vi "Test Next Shows Next Test to Run in Nested Test Suite.vi"(8 "error in (no error)":errorcluster, 11 "Test Case In":refnum<class "Test Suite Enumeration Test.lvclass">) -> (0 "error out":errorcluster, 3 "Test Case Out":refnum<class "Test Suite Enumeration Test.lvclass">)   [LabVIEW 2020, in "Test Suite Enumeration Test.lvclass"]
uses:
  Test Suite Enumeration Test.lvclass
  C:/Program Files (x86)/National Instruments/LabVIEW 2020/vi.lib/Astemes/LUnit/Test Case.lvclass
  Test Doubles/Test Case Test Double Child/Light Test Case Double.lvclass
  <vilib>/Astemes/LUnit/Test Case.lvclass/Test Case.ctl
  5f927c59-24be-4863-9429-5897c17c8022.vi
  <vilib>/Astemes/LUnit/Core/LUnit Test Case/Private/Append Pass Result.vi
  <vilib>/Astemes/LUnit/Core/LUnit Test Case/Private/Append Fail Result.vi
  5f927c59-24be-4863-9429-5897c17c8022.vi/9c5d11cd-9439-4240-a1ee-d9baace9c924.vi
  <vilib>/Astemes/LUnit/Core/LUnit Test Case/Private/Run In UI.vi
  <vilib>/Utility/error.llb/Clear Errors.vi
  source/Core/LUnit Test Suite/LUnit Test Suite.lvclass
  C:/git/astemes-lunit/source/Core/Runnable/Runnable.lvclass
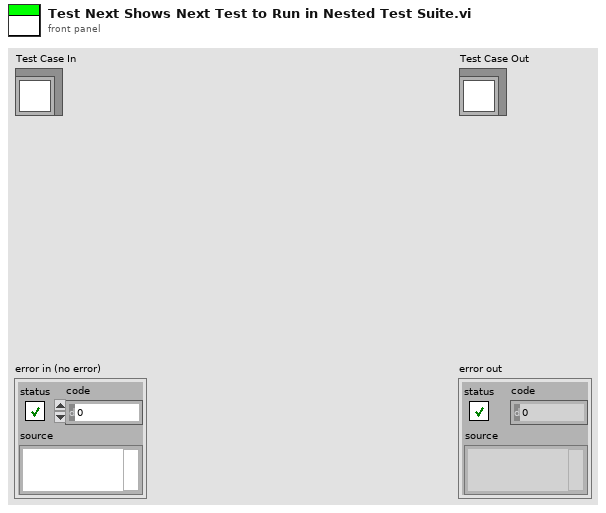
[diagram p1: front panel]
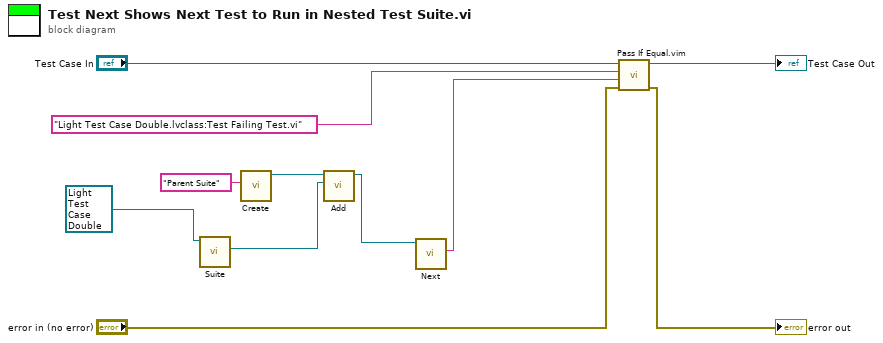
[diagram p0: block diagram]
diagram:
  n1 = call-dynamic "Suite.vi"("LUnit Test Case In"=refnum<class "Light Test Case Double.lvclass"> refnum ("Light Test Case Double.lvclass")) -> ("LUnit Test Suite Out"=w3:refnum<class "LUnit Test Suite.lvclass">)  [unwired: 8 in, 2 out]
  n2 = call "Create.vi"("Suite Name"="Parent Suite") -> ("LUnit Test Suite Out"=w4:refnum<class "LUnit Test Suite.lvclass">)  [unwired: 9 in, 1 out]
  n3 = call "Add.vi"("Runnable"=w3, "LUnit Test Suite In"=w4) -> ("LUnit Test Suite Out"=w2:refnum<class "LUnit Test Suite.lvclass">)  [unwired: 8 in, 1 out]
  n4 = call "Next.vi"("LUnit Test Suite In"=w2) -> ("Next Runnable"=w1:string)  [unwired: 8 in, 2 out]
  n5 = call "Pass If Equal.vim"("error in (no error)"="error in (no error)", "Actual"=w1, "Expected"="Light Test Case Double.lvclass:Test Failing Test.vi" ("Name"), "LUnit Test Case In"="Test Case In") -> ("error out"=→"error out":errorcluster, "LUnit Test Case Out"=→"Test Case Out":refnum<class "Test Suite Enumeration Test.lvclass">)  [unwired: 6 in]
